vi "Make DLL Param(Read Batch Profile Rsp).vi"(1 "Read Batch Profile Rsp":T2) -> (0 "pRsp":T1)   [LabVIEW 2014, in "Keyence LJ-V7000.lvlib"]
uses:
  Keyence LJ-V7000.lvlib
  Public/Clusters/Read Batch Profile Rsp.ctl
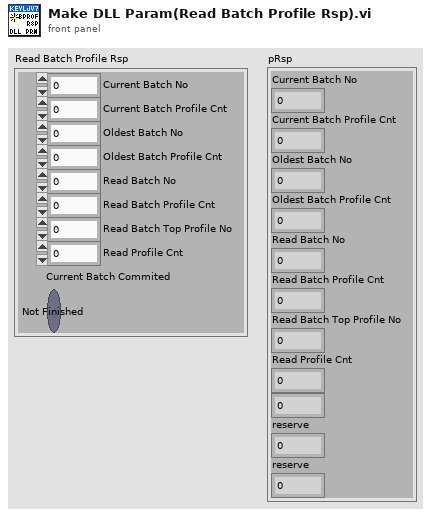
[diagram p1: front panel]
types:
  T1 = cluster{"Current Batch No":u32, "Current Batch Profile Cnt":u32, "Oldest Batch No":u32, "Oldest Batch Profile Cnt":u32, "Read Batch No":u32, "Read Batch Profile Cnt":u32, "Read Batch Top Profile No":u32, "Read Profile Cnt":u8, u8, "reserve":u8, "reserve":u8}
  T2 = typedef "Keyence LJ-V7000.lvlib/Read Batch Profile Rsp.ctl" = cluster{"Current Batch No":u32, "Current Batch Profile Cnt":u32, "Oldest Batch No":u32, "Oldest Batch Profile Cnt":u32, "Read Batch No":u32, "Read Batch Profile Cnt":u32, "Read Batch Top Profile No":u32, "Read Profile Cnt":u8, "Current Batch Commited":bool}
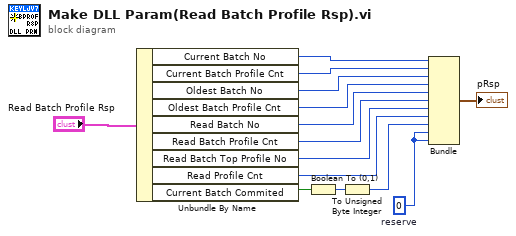
[diagram p0: block diagram]
diagram:
  w4 = u8 0  # reserve
  n1 = Unbundle By Name("Read Batch Profile Rsp") -> ("Current Batch No"=w14:u32, "Current Batch Profile Cnt"=w13:u32, "Oldest Batch No"=w12:u32, "Oldest Batch Profile Cnt"=w11:u32, "Read Batch No"=w9:u32, "Read Batch Profile Cnt"=w8:u32, "Read Batch Top Profile No"=w3:u32, "Read Profile Cnt"=w2:u8, "Current Batch Commited"=w6:bool)
  n2 = Boolean To (0,1)(Boolean=w6) -> (0, 1=w7:i16)
  n3 = To Unsigned Byte Integer(number=w7) -> (unsigned 8bit integer=w5:u8)
  n4 = Bundle("Current Batch No"=w14, "Current Batch Profile Cnt"=w13, "Oldest Batch No"=w12, "Oldest Batch Profile Cnt"=w11, "Read Batch No"=w9, "Read Batch Profile Cnt"=w8, "Read Batch Top Profile No"=w3, "Read Profile Cnt"=w2, w5, "reserve"=w4, "reserve"=w4) -> (→"pRsp":T1)  [unwired: 1 in]
